vi "User Events - Fire Timeout Event.vi"(8 "error in":errorcluster) -> (0 "error out":errorcluster)   [LabVIEW 2024, in "User Events.lvlib"]
uses:
  User Events.lvlib
  General Type Defs/FGV States.ctl
  General Type Defs/General Type Defs.lvlib
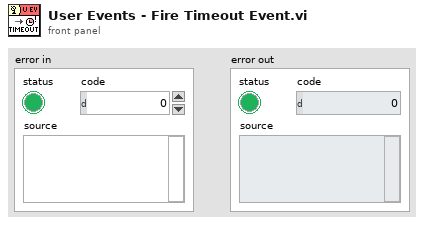
[diagram p1: front panel]
types:
  T1 = typedef "General Type Defs.lvlib/FGV States.ctl" = enum16{"Create", "Get", "Destroy"}
  T2 = typedef "General Type Defs.lvlib/User Events Cluster.ctl" = cluster{"STOP":refnum<user-event>, "Timeout":refnum<user-event>}
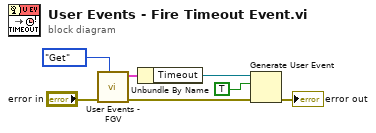
[diagram p0: block diagram]
diagram:
  n1 = call "User Events - FGV.vi"("FGV States"=FGV_States."Get", "error in"="error in") -> ("error out"=w2:errorcluster, "User Events Cluster"=w5:T2)  [unwired: 8 in]
  n2 = Unbundle By Name(w5) -> ("Timeout"=w4:refnum<user-event>)
  n3 = Generate User Event(user event=w4, event data cluster=TRUE ("event data"), error in=w2) -> (error out=→"error out":errorcluster)  [unwired: 1 in, 1 out]
